vi "TEST MMI Scaling (In SubPanel).vi"() -> ()   [LabVIEW 2013, in "IObject.lvclass"]
uses:
  IObject.lvclass
  <vilib>/Utility/miscctls.llb/LVRectTypeDef.ctl
  <vilib>/Utility/miscctls.llb/LVBoundsTypeDef.ctl
panel:
  in  "Boolean 2":bool
  in  "Boolean":bool
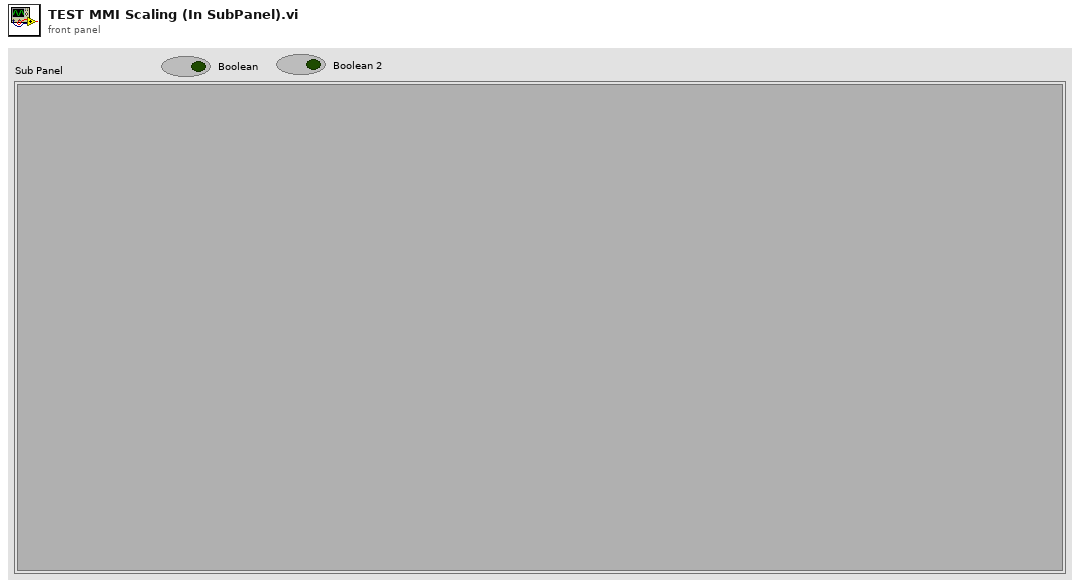
[diagram p1: front panel]
types:
  T1 = typedef "LVRectTypeDef.ctl" = cluster{"Left":i16, "Top":i16, "Right":i16, "Bottom":i16}
  T2 = typedef "LVBoundsTypeDef.ctl" = cluster{"Width":u32, "Height":u32}
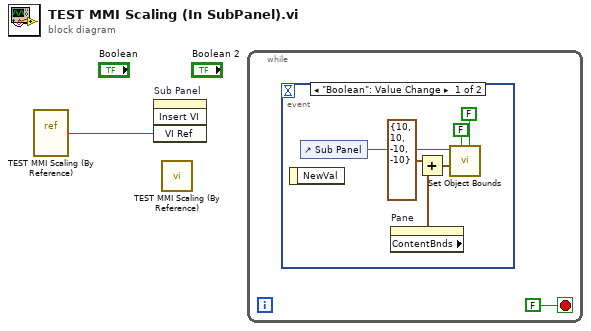
[diagram p0: block diagram]
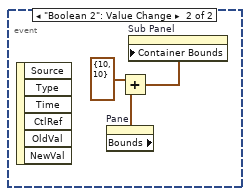
[diagram p2: hidden frame]
diagram:
  n1 = vi-ref "TEST MMI Scaling (By Reference).vi"() -> (w1:refnum<vi>)
  n2 = invoke on="Sub Panel" class="SubPnl" method="Insert VI"("VI Ref"=w1) -> ()  [unwired: 3 in, 4 out]
  n3 = call "TEST MMI Scaling (By Reference).vi"() -> ()  [unwired: 12 in]
  n4 = while {
    stop <- FALSE stop-if-true
    n5 = event shown="[0] \"Boolean\": Value Change" {
      selector: _ -> [_ _]
      dyn-events: _ -> [_ _]
      timeout: _ -> [_ _]
      event "Boolean": Value Change {
        n6 = event-data() -> ()  [unwired: 1 in, 1 out]
        n7 = control-ref of="Sub Panel"() -> (w3:refnum<vi>)
        n8 = property on="Pane" class="Pane"() -> ("ContentBnds"=w8:T1)  [unwired: 2 in, 2 out]
        n9 = Add(x=T1 {"Left"=10, "Top"=10, "Right"=-10, "Bottom"=-10}, y=w8) -> (x+y=w7:T1)
        n10 = call "Set Object Bounds.vi"("Resize Only? [F]"=FALSE ("Resize Only?"), "Position Only? [F]"=FALSE ("Position Only?"), "rect"=w7, "GObject"=w3) -> ()  [unwired: 6 in, 2 out]
      }
      event "Boolean 2": Value Change {
        n11 = event-data() -> ()  [unwired: 1 in, 6 out]
        n12 = property on="Pane" class="Pane"() -> ("Bounds"=w11:T2)  [unwired: 2 in, 2 out]
        n13 = Add(x=T2 {"Width"=10, "Height"=10}, y=w11) -> (x+y=w9:T2)
        n14 = property on="Sub Panel" class="SubPnl"("Container Bounds"=w9) -> ()  [unwired: 2 in, 2 out]
      }
    }
  }
